vi "QLV2.vi"(0 "Name":string, 5 "States":string, 7 "States[]":string[](array[string]), 11 "error in":errorcluster, 13 "Operation":T1) -> (4 "State Out":string, 15 "error out":errorcluster)   [LabVIEW 2020, in "CoffeeVending.lvlib"]
uses:
  CoffeeVending.lvlib
  TypeDef/QOperation.ctl
panel:
  # "Queue LV2"
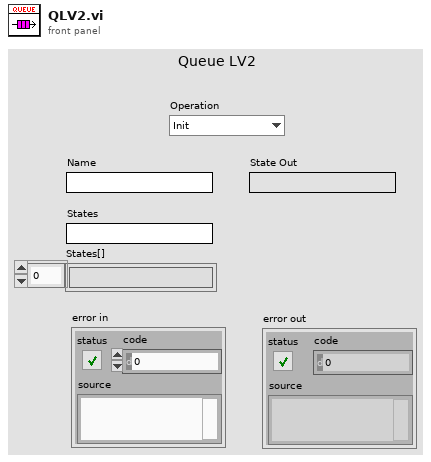
[diagram p1: front panel]
types:
  T1 = typedef "CoffeeVending.lvlib/QOperation.ctl" = enum16{"Init", "Enqueue", "Dequeue", "Enqueue N", "Enstack", "Release", "Flush"}
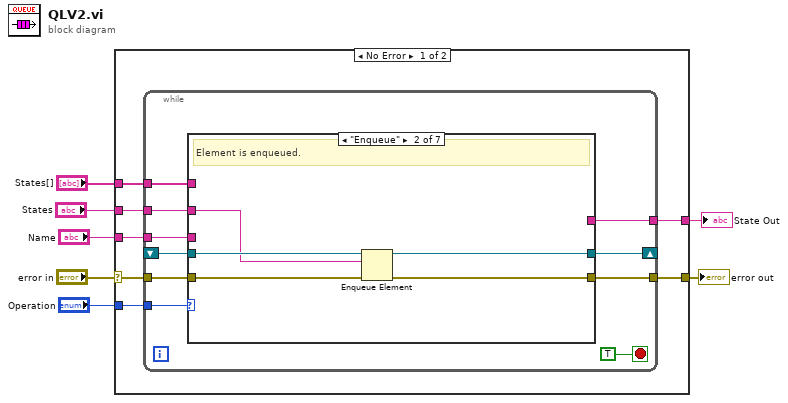
[diagram p0: block diagram]
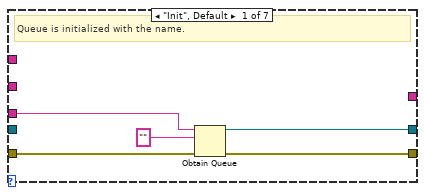
[diagram p2: hidden frame]
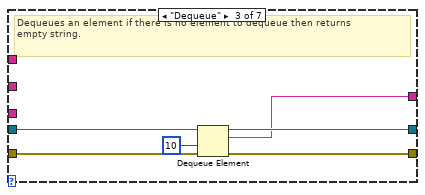
[diagram p3: hidden frame]
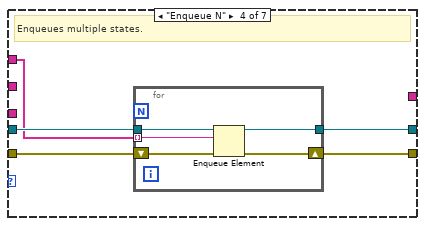
[diagram p4: hidden frame]
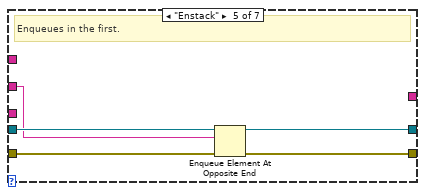
[diagram p5: hidden frame]
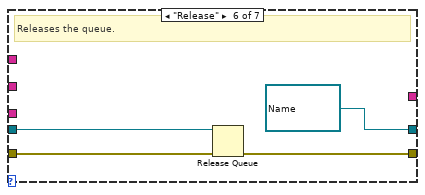
[diagram p6: hidden frame]
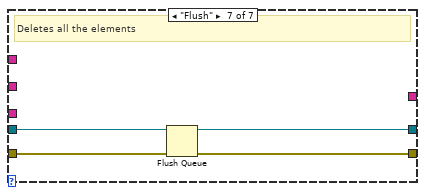
[diagram p7: hidden frame]
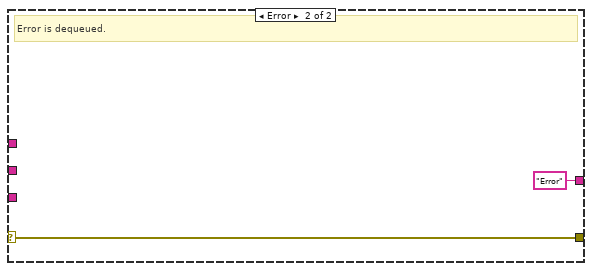
[diagram p8: hidden frame]
diagram:
  n1 = case shown="No Error" "error in" {
    selector: "error in" -> [w12 w64]
    tunnel: "Operation" -> [w14 _]
    tunnel: "Name" -> [w13 _]
    tunnel: [w11 w64] -> w1
    tunnel: "States" -> [w10 _]
    tunnel: [w9 "Error" ("Name")] -> w3
    tunnel: "States[]" -> [w8 _]
    frame No Error {
      n2 = while {
        tunnel: w14 -> [w23]
        tunnel: w13 -> [w22]
        tunnel: w12 -> [w21]
        tunnel: [w20] -> w11
        shift-right: [w19] -> _
        shift-left: _ -> [w18]
        tunnel: w10 -> [w17]
        tunnel: [w16] -> w9
        tunnel: w8 -> [w15]
        stop <- TRUE stop-if-true
        n3 = case shown="\"Enqueue\"" w23 {
          tunnel: w22 -> [w29 _ _ _ _ _ _]
          tunnel: w21 -> [w27 w34 w40 w45 w55 w59 w63]
          tunnel: [w26 w33 w39 w44 w54 w58 w62] -> w20
          tunnel: [w25 w31 w36 w42 w52 refnum<queue> refnum ("queue out") w60] -> w19
          tunnel: w18 -> [_ w32 w37 w43 w53 w57 w61]
          tunnel: w17 -> [_ w30 _ _ w51 _ _]
          tunnel: [_ _ w35 _ _ _ _] -> w16
          tunnel: w15 -> [_ _ _ w41 _ _ _]
          frame "Init", Default {
            # "Queue is initialized with the name."
            n4 = Obtain Queue(name (unnamed)=w29, element data type="" ("Name"), error in (no error)=w27) -> (queue out=w25:refnum<queue>, error out=w26:errorcluster)  [unwired: 2 in, 1 out]
          }
          frame "Enqueue" {
            # "Element is enqueued."
            n5 = Enqueue Element(queue=w32, element=w30, error in (no error)=w34) -> (queue out=w31:refnum<queue>, error out=w33:errorcluster)  [unwired: 1 in, 1 out]
          }
          frame "Dequeue" {
            # "Dequeues an element if there is no element to dequeue then returns\nempty string."
            n6 = Dequeue Element(queue=w37, timeout in ms (-1)=10, error in (no error)=w40) -> (queue out=w36:refnum<queue>, element=w35:string, error out=w39:errorcluster)  [unwired: 1 out]
          }
          frame "Enqueue N" {
            # "Enqueues multiple states."
            n7 = for {
              tunnel: w43 -> [w48]
              tunnel: [w47] -> w42
              shift-right: [w49] -> w44
              shift-left: w45 -> [w50]
              tunnel: w41 -> [w46] mode=indexing
              n8 = Enqueue Element(queue=w48, element=w46, error in (no error)=w50) -> (queue out=w47:refnum<queue>, error out=w49:errorcluster)  [unwired: 1 in, 1 out]
            }
          }
          frame "Enstack" {
            # "Enqueues in the first."
            n9 = Enqueue Element At Opposite End(queue=w53, element=w51, error in (no error)=w55) -> (queue out=w52:refnum<queue>, error out=w54:errorcluster)  [unwired: 1 in, 1 out]
          }
          frame "Release" {
            # "Releases the queue."
            n10 = Release Queue(queue=w57, error in (no error)=w59) -> (error out=w58:errorcluster)  [unwired: 1 in, 2 out]
          }
          frame "Flush" {
            # "Deletes all the elements"
            n11 = Flush Queue(queue=w61, error in (no error)=w63) -> (queue out=w60:refnum<queue>, error out=w62:errorcluster)  [unwired: 1 out]
          }
        }
      }
    }
    frame Error {
      # "Error is dequeued."
    }
  }
  "State Out" <- w3
  "error out" <- w1
